vi "SquareRoot.vi"() -> ()   [LabVIEW 2018]
panel:
  out "Square root value":dbl
  in  "Number":dbl
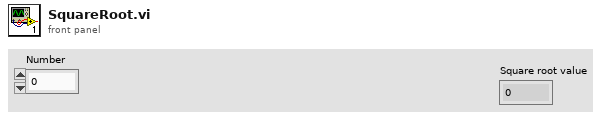
[diagram p1: front panel]
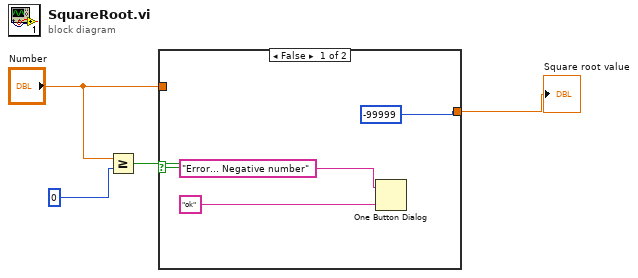
[diagram p0: block diagram]
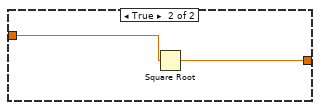
[diagram p2: hidden frame]
diagram:
  n1 = Greater Or Equal?(x="Number", y=0) -> (x >= y?=w3:bool)
  n2 = case shown="False" w3 {
    tunnel: "Number" -> [_ w9]
    tunnel: [-99999 w8] -> w4
    frame False {
      n3 = One Button Dialog(message="Error... Negative number", button name ("OK")="ok") -> ()  [unwired: 1 out]
    }
    frame True {
      n4 = Square Root(x=w9) -> (sqrt(x)=w8:dbl)
    }
  }
  "Square root value" <- w4
